vi "Scalar JSON text to Variant.vi"(6 "Type":T1, 8 "error in (no error)":errorcluster, 9 "Variant (Data Type)":variant, 10 "Offset":i32, 11 "JSON":string) -> (0 "error out":errorcluster, 1 "Variant out":variant)   [LabVIEW 2017, in "JSONtext.lvlib"]
uses:
  JSONtext.lvlib
  <vilib>/Utility/Data Type/Type Definitions/Data Type.ctl
  <vilib>/Utility/Data Type/Type Definitions/Refnum Type.ctl
  Advance past String.vi
  String Subset.vi
  support/Strip Quotes and Unescape.vi
  support/Get Number Text.vi
  NaN or null to Integer ERROR.vi
  Advance past Number.vi
  support/Unescape JSON string.vi
  Parsing Error in converting to LabVIEW type.vi
  <vilib>/JDP Science/JDP Science Common Utilities/Timestamp/Text to Timestamp.vi
  <vilib>/Utility/Data Type/NI_Data Type.lvlib
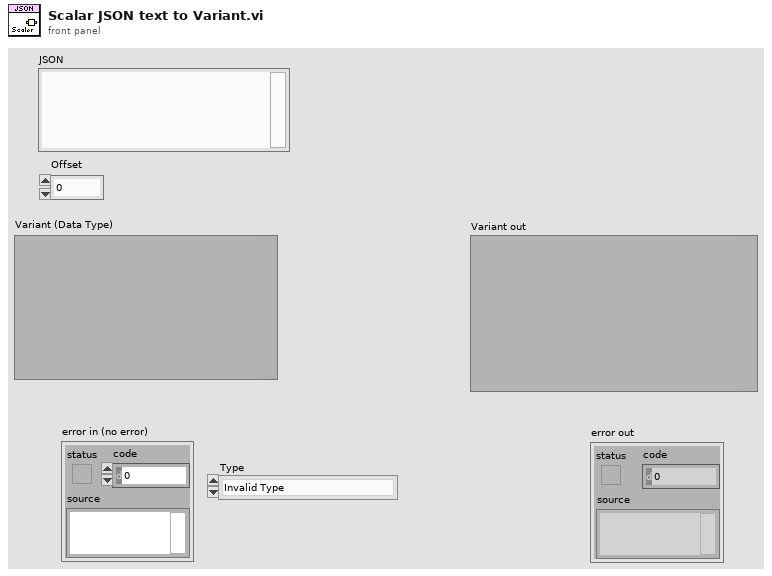
[diagram p1: front panel]
types:
  T1 = typedef "NI_Data Type.lvlib/Data Type.ctl" = enum8{"Invalid Type", "Void", "I8", "I16", "I32", "I64", "U8", "U16", "U32", "U64", "Single Float", "Double Float", "Extended Float", "Single Complex", "Double Complex", "Extended Complex", "Enum U8", "Enum U16", "Enum U32", "Enum U64", "Single Float With Unit", "Double Float With Unit", "Extended Float With Unit", "Single Complex with Unit", "Double Complex with Unit", "Extended Complex with Unit", "Boolean", "String", "Path", "Picture", "Tag", "Array", "Cluster", "Variant", "LV Variant", "Waveform", "Timestamp", "Digital Waveform", "Digital Data", "ExpressData", "Refnum", "External Data", "VI", "Poly VI", "LabVIEW Class Instance", "Fixed Point"}
  T2 = typedef "JSONtext.lvlib/Parsing State.ctl" = enum16{"Parser Error", "Object", "Array", "String", "Number/Other", "Leading Whitespace", "Object end", "Array end", "Value end"}
  T3 = typedef "NI_Data Type.lvlib/Refnum Type.ctl" = enum16{"NotARefnum", "UnknownRefnum", "Generic", "Datalog", "ByteStream", "Device", "Occurence", "TCPNetConnection", "Auto", "Menu", "Imaq", "Hardware", "DataSocket", "Visa", "IVI", "UDPNetConnection", "Notifier", "Queue", "Irda", "EventReg", "DotNet", "UserEvent", "Callback", "UNUSED_EMPTY_POSITION", "BlueToothNetConnection", "LVObjApp", "LVObjVI", "LVObjUnknown", "GenericClass", "UserDefinedRefnumTag", "DataValue", "RT FIFO", "TDMS File"}
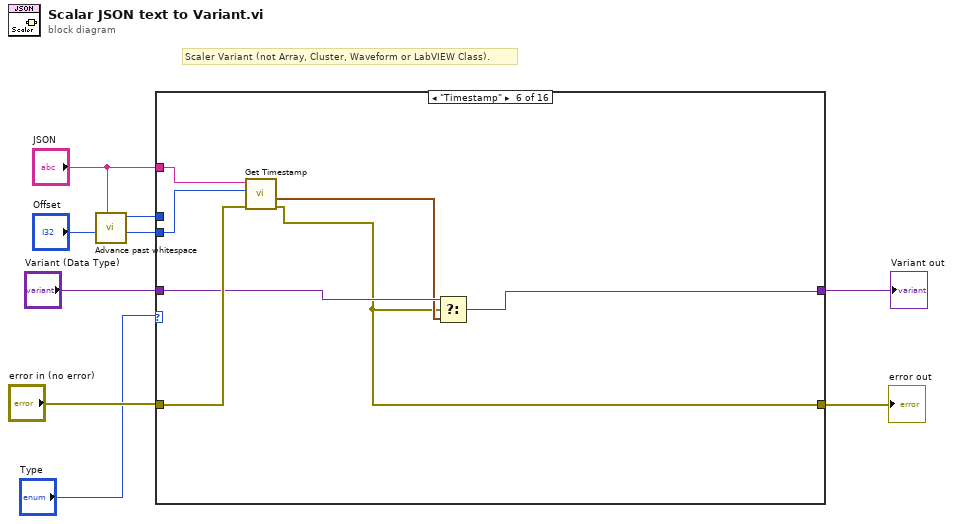
[diagram p0: block diagram]
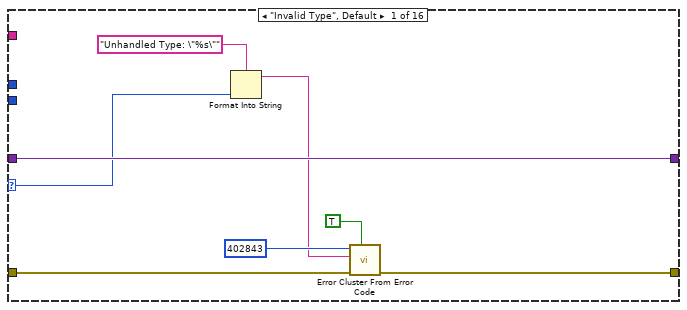
[diagram p2: hidden frame]
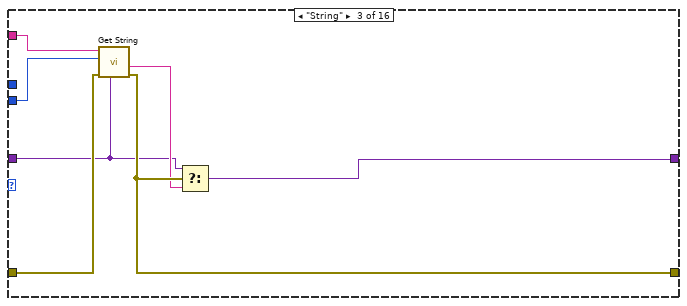
[diagram p4: hidden frame]
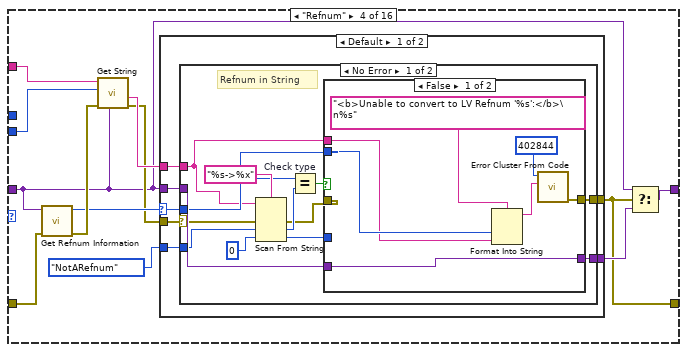
[diagram p5: hidden frame]
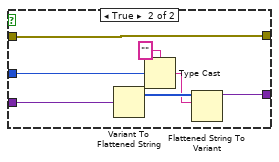
[diagram p6: hidden frame]
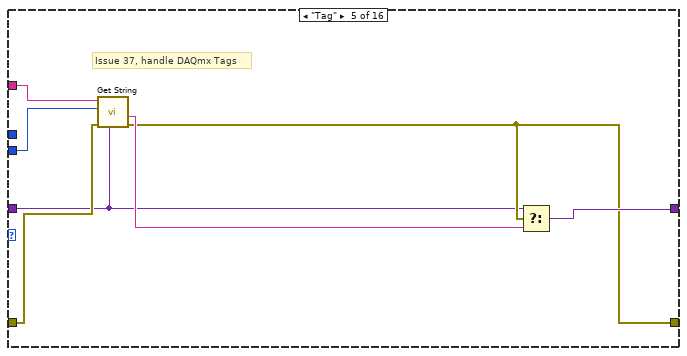
[diagram p9: hidden frame]
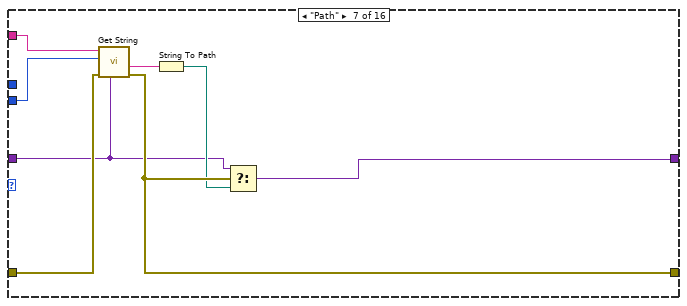
[diagram p10: hidden frame]
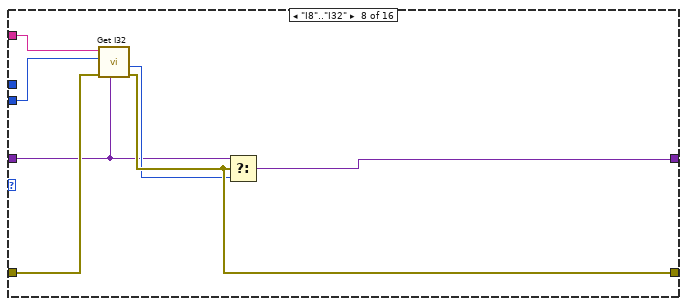
[diagram p11: hidden frame]
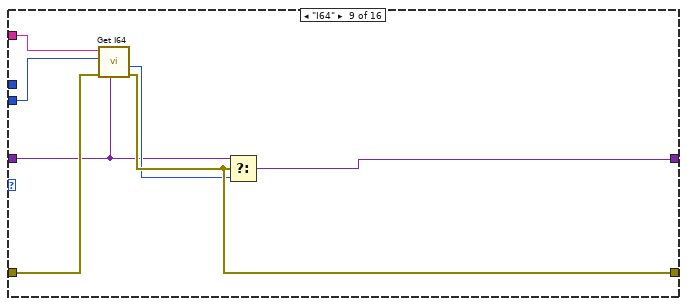
[diagram p12: hidden frame]
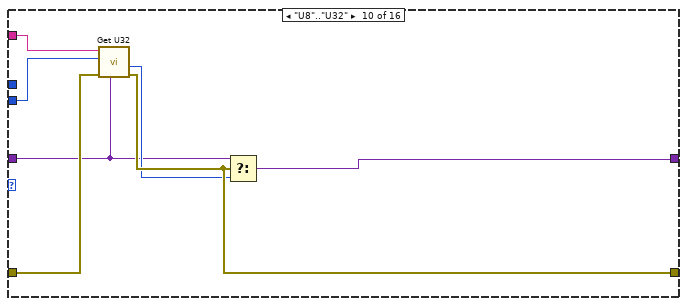
[diagram p13: hidden frame]
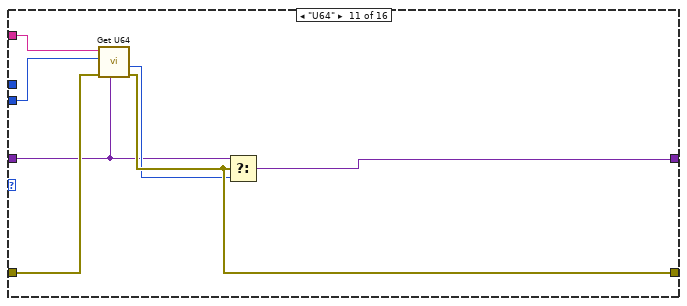
[diagram p14: hidden frame]
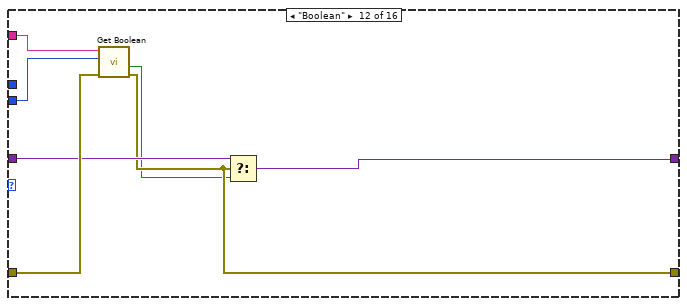
[diagram p15: hidden frame]
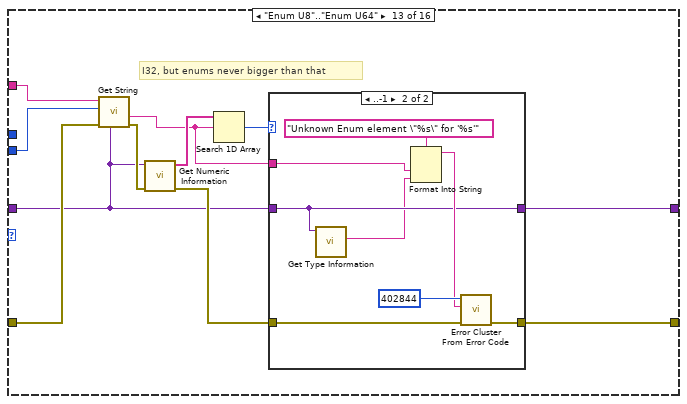
[diagram p16: hidden frame]
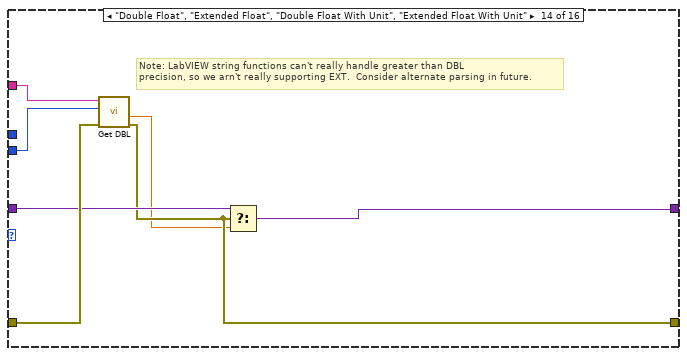
[diagram p18: hidden frame]
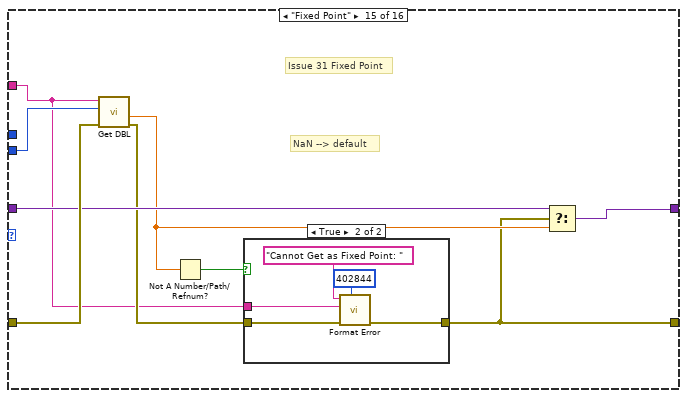
[diagram p19: hidden frame]
diagram:
  # "Scaler Variant (not Array, Cluster, Waveform or LabVIEW Class)."
  n1 = call "Advance past whitespace.vi"("JSON"="JSON", "Offset"="Offset") -> ("Offset of first non-whitespace"=w5:i32, "Parser State"=w3:T2)  [unwired: 8 in]
  n2 = case shown="\"Timestamp\"" "Type" {
    selector: "Type" -> [w12 _ _ _ _ _ _ _ _ _ _ _ _ _ _ _]
    tunnel: "Variant (Data Type)" -> [w16 w18 w20 w27 w76 w86 w90 w98 w105 w112 w119 w130 w133 w158 w167 w180]
    tunnel: "JSON" -> [_ _ w25 w37 w81 w88 w96 w100 w107 w114 w121 w127 w141 w155 w163 w177]
    tunnel: [w15 w19 w22 w29 w77 w83 w93 w101 w108 w115 w122 w128 w137 w156 w161 w178] -> w8
    tunnel: "error in (no error)" -> [w17 w19 w24 w35 w79 w87 w95 w103 w110 w117 w124 w131 w142 w159 w168 w181]
    tunnel: w5 -> [_ _ w26 w38 w82 w89 w97 w104 w111 w118 w125 w132 w143 w160 w169 w182]
    tunnel: [w16 w18 w23 w36 w80 w85 w94 w102 w109 w116 w123 w129 w138 w157 w166 w179] -> w7
    tunnel: w3 -> [_ _ _ _ _ _ _ _ _ _ _ _ _ _ _ _]
    frame "Invalid Type", Default {
      n3 = Format Into String(format string="Unhandled Type: \"%s\"", w12) -> (resulting string=w10:string)  [unwired: 2 in, 1 out]
      n4 = call <vilib>:"Error Cluster From Error Code.vi"("show call chain? (False)"=TRUE, "error in (no error)"=w17, "error message (\"\")"=w10, "error code (0)"=402843) -> ("error out"=w15:errorcluster)  [unwired: 5 in]
    }
    frame "Void" {
      # "Empty Variant: #ToDo Variant Attributes?"
    }
    frame "String" {
      n5 = call "Get String.vi"("LV Type"=w20, "error in (no error)"=w24, "Offset"=w26, "JSON"=w25) -> ("error out"=w22:errorcluster, "String"=w21:string)  [unwired: 5 in, 1 out]
      n6 = Select(t=w20, s=w22, f=w21) -> (s? t:f=w23:variant)
    }
    frame "Refnum" {
      n7 = call <vilib>:"Get Refnum Information.vi"("error in (no error)"=w35, "Variant"=w27) -> ("error out"=w34:errorcluster, "Reference Type"=w33:T3)  [unwired: 6 in, 2 out]
      n8 = call "Get String.vi"("LV Type"=w27, "error in (no error)"=w34, "Offset"=w38, "JSON"=w37) -> ("error out"=w30:errorcluster, "String"=w31:string)  [unwired: 5 in, 1 out]
      n9 = case shown="Default" w33 {
        selector: w33 -> [w39 _]
        tunnel: [w44 w75] -> w32
        tunnel: w31 -> [w41 w75]
        tunnel: w27 -> [w45 _]
        tunnel: w30 -> [w43 w74]
        tunnel: [w42 w74] -> w29
        tunnel: Refnum_Type."NotARefnum" ("Reference Type") -> [w40 _]
        frame Default {
          n10 = case shown="No Error" w43 {
            selector: w43 -> [w53 w73]
            tunnel: w45 -> [w58 _]
            tunnel: [w57 _] -> w44
            tunnel: [w48 w73] -> w42
            tunnel: w41 -> [w46 _]
            tunnel: w40 -> [w52 _]
            tunnel: w39 -> [w47 _]
            frame No Error {
              # "Refnum in String"
              n11 = Scan From String(format string="%s->%x", input string=w46, error in=w53, default 1=w52, default 2=u32 0) -> (error out=w49:errorcluster, output 1=w51:T3, output 2=w54:u32)  [unwired: 1 in, 2 out]
              n12 = Equal? "Check type"(x=w47, y=w51) -> (x = y?=w50:bool)
              n13 = case shown="False" w50 {
                tunnel: w58 -> [w65 w70]
                tunnel: [w65 w69] -> w57
                tunnel: w54 -> [_ w67]
                tunnel: w49 -> [_ w66]
                tunnel: [w64 w66] -> w48
                tunnel: w47 -> [w60 _]
                tunnel: w46 -> [w59 _]
                frame False {
                  n14 = Format Into String(format string="<b>Unable to convert to LV Refnum '%s':</b>\n%s", w60, w59) -> (resulting string=w62:string)  [unwired: 2 in, 1 out]
                  n15 = call "Error Cluster From Code.vi"("error message (\"\")"=w62, "error code (402840+)"=402844) -> ("error out"=w64:errorcluster)  [unwired: 7 in]
                }
                frame True {
                  n16 = Variant To Flattened String(Variant=w70) -> (1:w72:i16[])  [unwired: 1 out]
                  n17 = Type Cast(type="", x=w67) -> (*(type *) &x=w71:string)
                  n18 = Flattened String To Variant(6:w71, 7:w72) -> (3:w69:variant)  [unwired: 1 in, 1 out]
                }
              }
            }
            frame Error {
            }
          }
        }
        frame "Visa", "IVI", "UserDefinedRefnumTag" {
        }
      }
      n19 = Select(t=w27, s=w29, f=w32) -> (s? t:f=w36:variant)
    }
    frame "Tag" {
      # "Issue 37, handle DAQmx Tags"
      n20 = call "Get String.vi"("LV Type"=w76, "error in (no error)"=w79, "Offset"=w82, "JSON"=w81) -> ("error out"=w77:errorcluster, "String"=w78:string)  [unwired: 5 in, 1 out]
      n21 = Select(t=w76, s=w77, f=w78) -> (s? t:f=w80:variant)
    }
    frame "Timestamp" {
      n22 = call "Get Timestamp.vi"("error in (no error)"=w87, "Offset"=w89, "JSON"=w88) -> ("error out"=w83:errorcluster, "Timestamp"=w84:timestamp)  [unwired: 6 in, 1 out]
      n23 = Select(t=w86, s=w83, f=w84) -> (s? t:f=w85:variant)
    }
    frame "Path" {
      n24 = call "Get String.vi"("LV Type"=w90, "error in (no error)"=w95, "Offset"=w97, "JSON"=w96) -> ("error out"=w93:errorcluster, "String"=w91:string)  [unwired: 5 in, 1 out]
      n25 = String To Path(string=w91) -> (path=w92:path)
      n26 = Select(t=w90, s=w93, f=w92) -> (s? t:f=w94:variant)
    }
    frame "I8".."I32" {
      n27 = call "Get I32.vi"("LV Type"=w98, "error in (no error)"=w103, "Offset"=w104, "JSON"=w100) -> ("error out"=w101:errorcluster, "Number"=w99:i32)  [unwired: 5 in, 1 out]
      n28 = Select(t=w98, s=w101, f=w99) -> (s? t:f=w102:variant)
    }
    frame "I64" {
      n29 = call "Get I64.vi"("LV Type"=w105, "error in (no error)"=w110, "Offset"=w111, "JSON"=w107) -> ("error out"=w108:errorcluster, "Number"=w106:i64)  [unwired: 5 in, 1 out]
      n30 = Select(t=w105, s=w108, f=w106) -> (s? t:f=w109:variant)
    }
    frame "U8".."U32" {
      n31 = call "Get U32.vi"("LV Type"=w112, "error in (no error)"=w117, "Offset"=w118, "JSON"=w114) -> ("error out"=w115:errorcluster, "Number"=w113:u32)  [unwired: 5 in, 1 out]
      n32 = Select(t=w112, s=w115, f=w113) -> (s? t:f=w116:variant)
    }
    frame "U64" {
      n33 = call "Get U64.vi"("LV Type"=w119, "error in (no error)"=w124, "Offset"=w125, "JSON"=w121) -> ("error out"=w122:errorcluster, "Number"=w120:u64)  [unwired: 5 in, 1 out]
      n34 = Select(t=w119, s=w122, f=w120) -> (s? t:f=w123:variant)
    }
    frame "Boolean" {
      n35 = call "Get Boolean.vi"("error in (no error)"=w131, "Offset"=w132, "JSON"=w127) -> ("error out"=w128:errorcluster, "Boolean"=w126:bool)  [unwired: 6 in, 1 out]
      n36 = Select(t=w130, s=w128, f=w126) -> (s? t:f=w129:variant)
    }
    frame "Enum U8".."Enum U64" {
      # "I32, but enums never bigger than that"
      n37 = call "Get String.vi"("LV Type"=w133, "error in (no error)"=w142, "Offset"=w143, "JSON"=w141) -> ("error out"=w135:errorcluster, "String"=w136:string)  [unwired: 5 in, 1 out]
      n38 = call <vilib>:"Get Numeric Information.vi"("error in (no error)"=w135, "Variant"=w133) -> ("error out"=w134:errorcluster, "Enum Names"=w139:string[])  [unwired: 6 in, 2 out]
      n39 = Search 1D Array(1D array=w139, element=w136) -> (index of element=w140:i32)  [unwired: 1 in]
      n40 = case shown="..-1" w140 {
        selector: w140 -> [w144 _]
        tunnel: [w144 w148] -> w138
        tunnel: w133 -> [_ w148]
        tunnel: w134 -> [w145 w151]
        tunnel: [w145 w153] -> w137
        tunnel: w136 -> [_ w146]
        frame 0.. {
        }
        frame ..-1 {
          n41 = call <vilib>:"Get Type Information.vi"("Variant"=w148) -> ("Name"=w147:string)  [unwired: 6 in, 4 out]
          n42 = Format Into String(format string="Unknown Enum element \"%s\" for '%s'", w146, w147) -> (resulting string=w149:string)  [unwired: 2 in, 1 out]
          n43 = call <vilib>:"Error Cluster From Error Code.vi"("error in (no error)"=w151, "error message (\"\")"=w149, "error code (0)"=402844) -> ("error out"=w153:errorcluster)  [unwired: 6 in]
        }
      }
    }
    frame "Double Float", "Extended Float", "Double Float With Unit", "Extended Float With Unit" {
      # "Note: LabVIEW string functions can't really handle greater than DBL\nprecision, so we arn't really supporting EXT.  Consider alternate parsing in future."
      n44 = call "Get DBL.vi"("error in (no error)"=w159, "Offset"=w160, "JSON"=w155) -> ("error out"=w156:errorcluster, "Number"=w154:dbl)  [unwired: 6 in, 1 out]
      n45 = Select(t=w158, s=w156, f=w154) -> (s? t:f=w157:variant)
    }
    frame "Fixed Point" {
      # "NaN --> default"
      # "Issue 31 Fixed Point"
      n46 = call "Get DBL.vi"("error in (no error)"=w168, "Offset"=w169, "JSON"=w163) -> ("error out"=w164:errorcluster, "Number"=w165:dbl)  [unwired: 6 in, 1 out]
      n47 = Not A Number/Path/Refnum?(number/path/refnum=w165) -> (NaN/Path/Refnum?=w162:bool)
      n48 = case shown="True" w162 {
        tunnel: w164 -> [w170 w175]
        tunnel: [w170 w174] -> w161
        tunnel: w163 -> [_ w171]
        frame False {
        }
        frame True {
          n49 = call "Format Error.vi"("error code (402842)"=402844, "error in (no error)"=w175, "message part 2"=w171, "error message"="Cannot Get as Fixed Point: " ("format string")) -> ("error out"=w174:errorcluster)  [unwired: 7 in]
        }
      }
      n50 = Select(t=w167, s=w161, f=w165) -> (s? t:f=w166:variant)
    }
    frame "Single Float", "Single Float With Unit" {
      n51 = call "Get SGL.vi"("error in (no error)"=w181, "Offset"=w182, "JSON"=w177) -> ("error out"=w178:errorcluster, "Number"=w176:sgl)  [unwired: 6 in, 1 out]
      n52 = Select(t=w180, s=w178, f=w176) -> (s? t:f=w179:variant)
    }
  }
  "Variant out" <- w7
  "error out" <- w8
